vi "AI_snake.vi"() -> ()   [LabVIEW 2020]
uses:
  Typedef/Snake_states.ctl
panel:
  in  "speed":dbl=700.0 format="%#_13g"
  in  "level":dbl(slide) scale=1.0..5.0
  out "Stop Variable":bool
  out "Score":i32
  out "Snake Field":u32[][](array[colorbox])=[[0, 0, 0, 0, 0, 0, 0, 0, 0, 0, 0, 0, 0, 0, 0, 0, 0, 0, 0, 0, 0, 0, 0, 0, 0, 0, 0], [0, 0, 0, 0, 0, 0, 0, 0, 0, 0, 0, 0, 0, 0, 0, 0, 0, 0, 0, 0, 0, 0, 0, 0, 0, 0, 0], [0, 0, 0, 3622, 0, 0, 0, 0, 0, 0, 0, 0, 0, 0, 0, 0, 0, 0, 0, 0, 0, 0, 0, 0, 0, 0, 0], [0, 0, 0, 0, 0, 0, 0, 0, 0, 0, 0, 0, 0, 0, 0, 0, 0, 0, 0, 0, 0, 0, 0, 0, 0, 0, 0], [0, 0, 0, 0, 0, 0, 0, 0, 0, 0, 0, 0, 0, 0, 0, 0, 0, 0, 0, 0, 0, 0, 0, 0, 0, 0, 0], [0, 0, 0, 0, 0, 0, 0, 0, 0, 0, 0, 0, 0, 0, 0, 0, 0, 0, 0, 0, 0, 0, 0, 0, 0, 0, 0], [0, 0, 0, 0, 0, 0, 0, 0, 0, 0, 0, 0, 0, 0, 0, 0, 0, 0, 0, 0, 0, 0, 0, 0, 0, 0, 0], [0, 0, 0, 0, 0, 0, 0, 0, 0, 0, 0, 0, 0, 0, 0, 0, 0, 0, 0, 0, 0, 0, 0, 0, 0, 0, 0], [0, 0, 0, 0, 0, 0, 0, 0, 0, 0, 0, 0, 0, 0, 0, 0, 0, 0, 0, 0, 0, 0, 0, 0, 0, 0, 0], [0, 0, 0, 0, 0, 0, 0, 0, 0, 0, 0, 0, 0, 0, 0, 0, 0, 0, 0, 0, 0, 0, 0, 0, 0, 0, 0], [0, 0, 0, 0, 0, 0, 0, 0, 0, 0, 0, 0, 0, 0, 0, 0, 0, 0, 0, 0, 0, 0, 0, 0, 0, 0, 0], [0, 0, 0, 0, 0, 0, 0, 0, 0, 0, 0, 0, 0, 0, 0, 0, 0, 0, 0, 0, 0, 0, 0, 0, 0, 0, 0], [0, 0, 0, 0, 0, 0, 0, 0, 0, 0, 0, 0, 0, 0, 0, 0, 0, 0, 0, 0, 0, 0, 0, 0, 0, 0, 0], [0, 0, 0, 0, 0, 0, 0, 0, 0, 0, 0, 0, 0, 0, 0, 0, 0, 0, 0, 0, 0, 0, 0, 0, 0, 0, 0], [0, 0, 0, 0, 0, 0, 0, 0, 0, 0, 0, 0, 0, 0, 0, 0, 0, 0, 0, 0, 0, 0, 0, 0, 0, 0, 0], [0, 0, 0, 0, 0, 0, 0, 0, 0, 0, 0, 0, 0, 0, 0, 0, 0, 0, 0, 0, 0, 0, 0, 0, 0, 0, 0], [0, 0, 0, 0, 0, 0, 0, 0, 0, 0, 0, 0, 0, 0, 0, 0, 0, 0, 0, 0, 0, 0, 0, 0, 0, 0, 0], [0, 0, 0, 0, 0, 0, 0, 0, 0, 0, 0, 0, 0, 0, 0, 0, 0, 0, 0, 0, 0, 0, 0, 0, 0, 0, 0], [0, 0, 0, 0, 0, 0, 0, 0, 0, 0, 0, 0, 0, 0, 0, 0, 0, 0, 0, 0, 0, 0, 0, 0, 0, 0, 0], [0, 0, 0, 0, 0, 0, 0, 0, 0, 0, 0, 0, 0, 0, 0, 0, 0, 0, 0, 0, 0, 0, 0, 0, 0, 0, 0]]
  out "Y Direction":i32
  out "X Direction":i32
  in  "Stop":bool
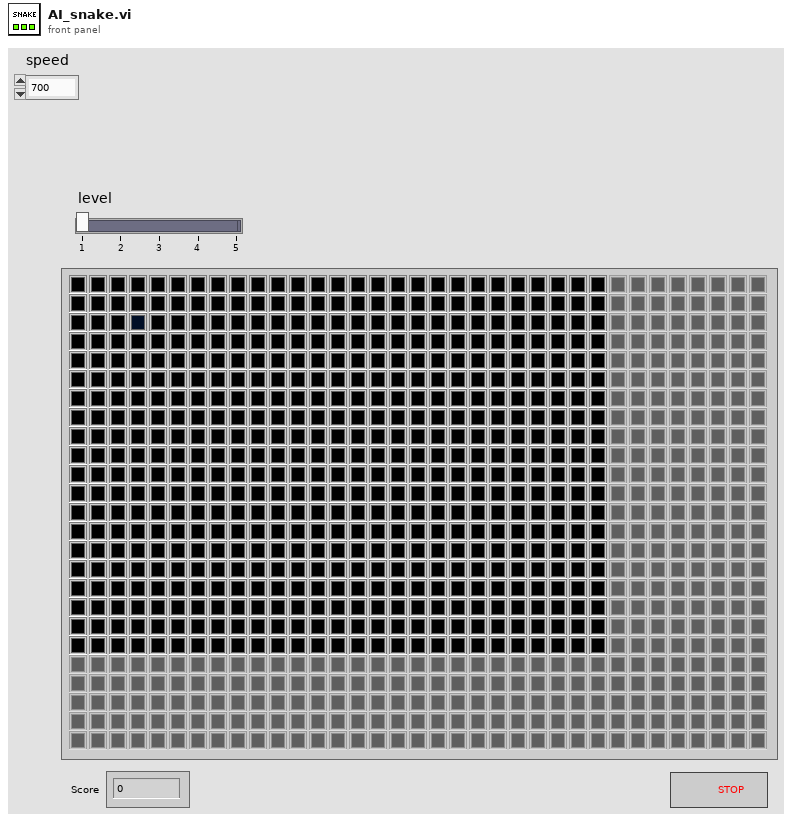
[diagram p1: front panel]
types:
  T1 = typedef "Snake_states.ctl" = enum16{"Initialize", "Start game", "Wait for user to press button", "Stop"}
  T2 = typedef "eventvkey.ctl" = enum16{"ASCII", "Enter", "Return", "Shift", "Ctrl", "Alt", "Cmd", "Opt", "Caps", "NumLock", "Clear", "Break", "Up", "Down", "Left", "Right", "Insert", "Delete", "Home", "End", "PageUp", "PageDown", "Escape", "Help", "Pause", "ScrollLock", "F1", "F2", "F3", "F4", "F5", "F6", "F7", "F8", "F9", "F10", "F11", "F12", "F13", "F14", "F15", "F16", "F17", "F18", "F19", "F20", "F21", "F22", "F23", "F24", "Play", "VolumeUp", "VolumeDown", "Mute", "Two Byte Char"}
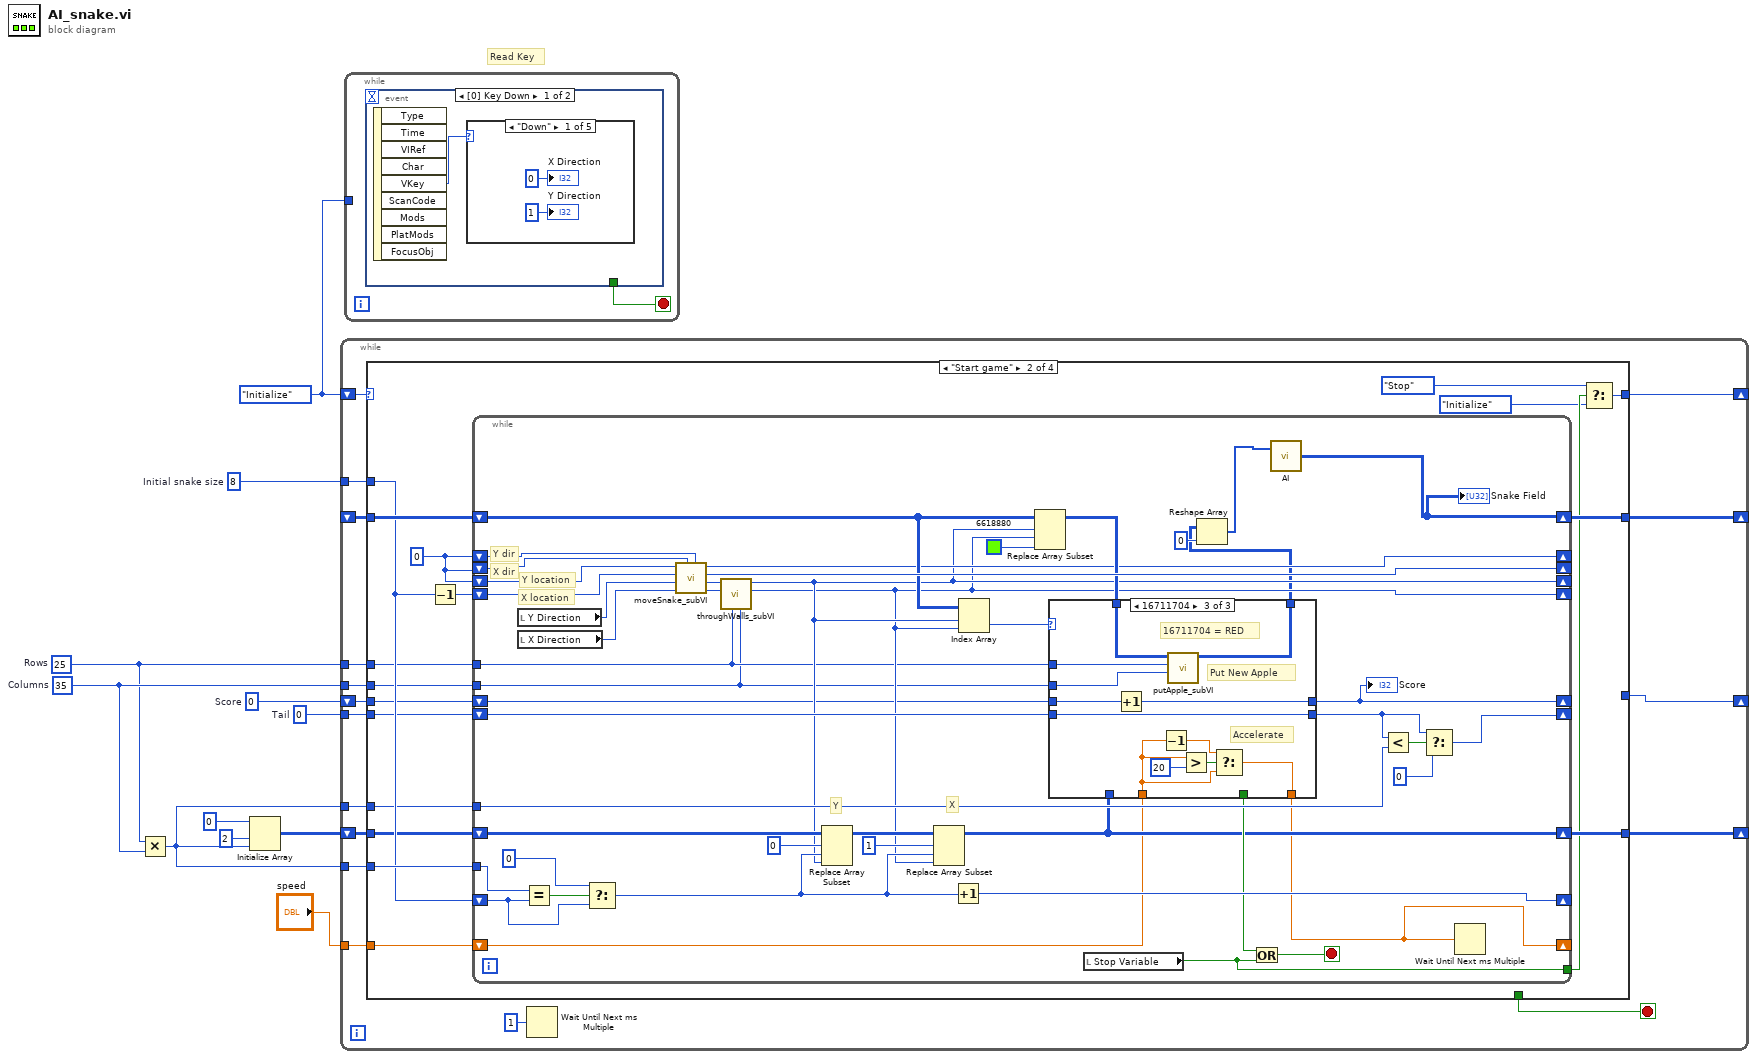
[diagram p0: block diagram]
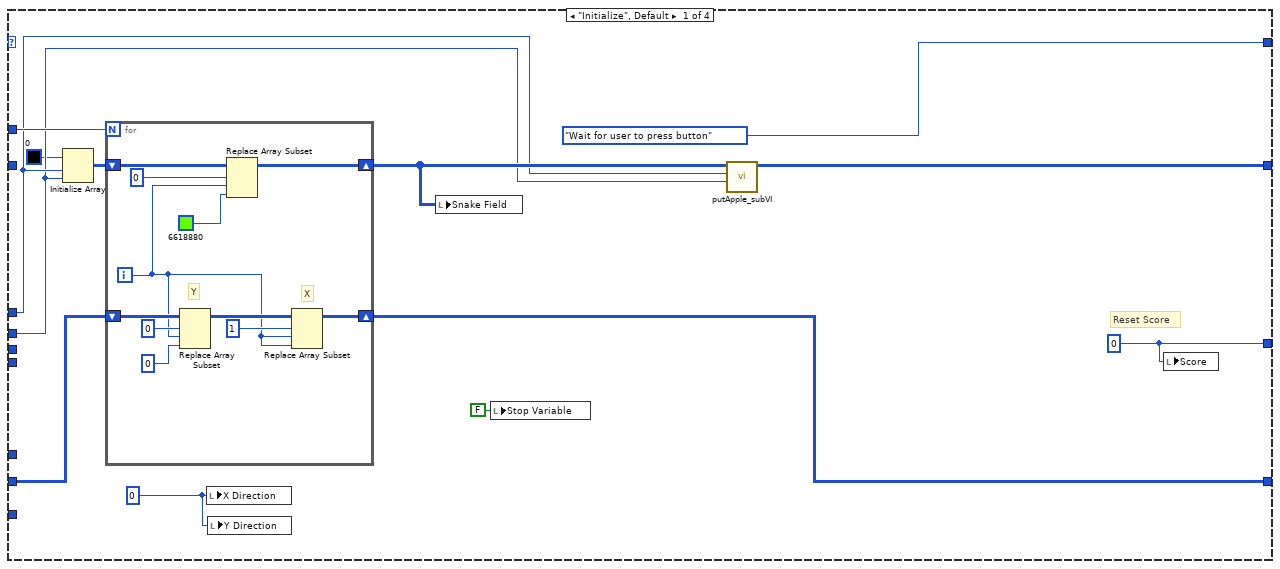
[diagram p2: hidden frame]
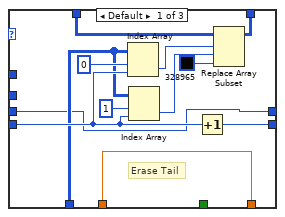
[diagram p3: hidden frame]
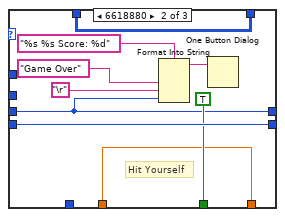
[diagram p4: hidden frame]
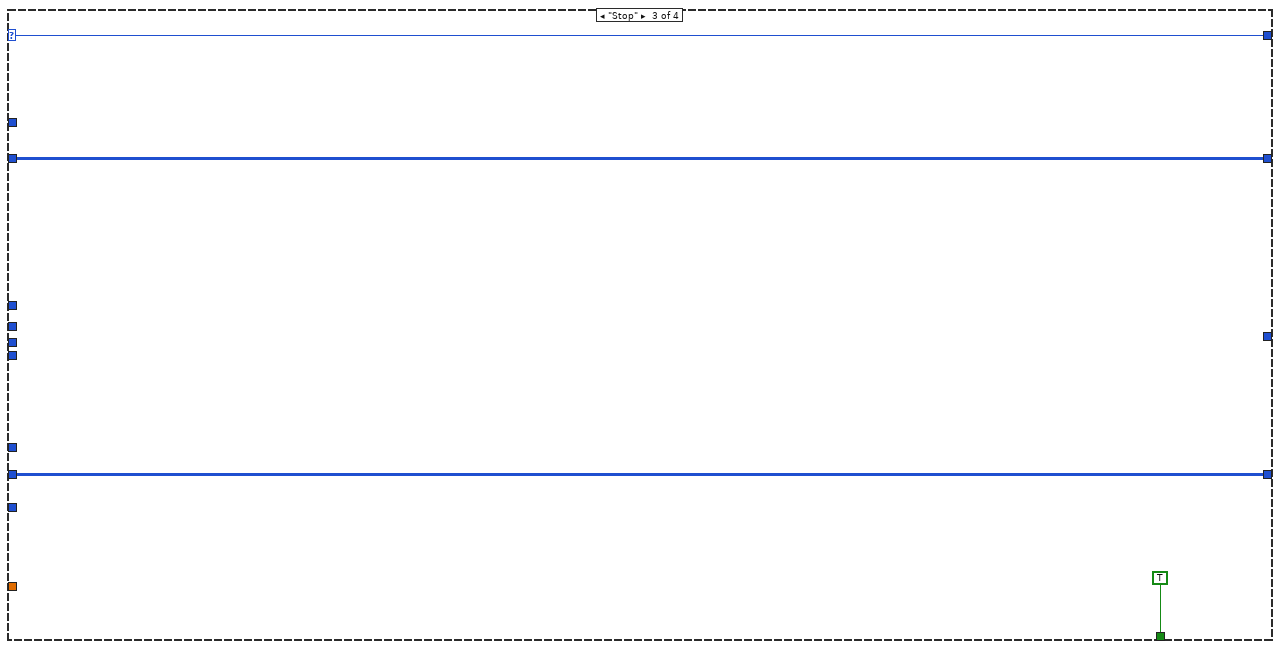
[diagram p5: hidden frame]
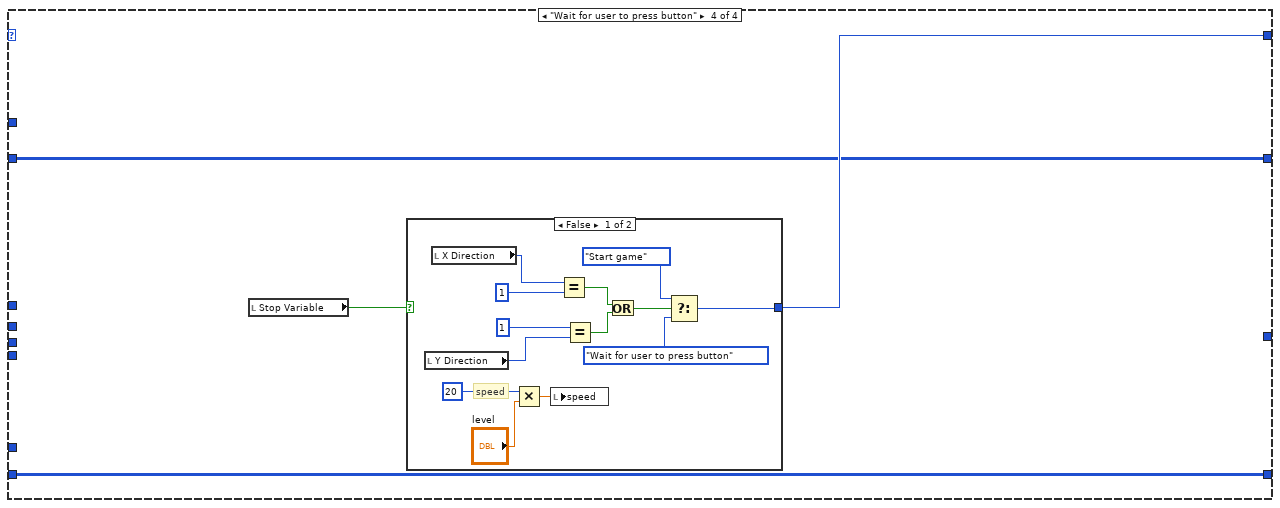
[diagram p6: hidden frame]
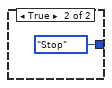
[diagram p7: hidden frame]
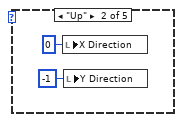
[diagram p8: hidden frame]
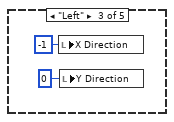
[diagram p9: hidden frame]
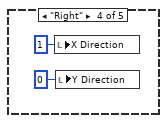
[diagram p10: hidden frame]
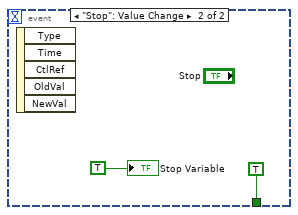
[diagram p12: hidden frame]
diagram:
  w2 = 0  # Score
  w6 = 0  # Tail
  w10 = 8  # Initial snake size
  w5 = 35  # Columns
  w4 = 25  # Rows
  w11 = Snake_states."Initialize"
  # "Read Key"
  n1 = Multiply(x=w4, y=w5) -> (x*y=w3:i32)
  n2 = Initialize Array(0 ("element"), 2 ("dimension size"), w3) -> (w7:i32[][])
  n3 = while {
    shift-right: [w27] -> _
    shift-left: w11 -> [w28]
    tunnel: w3 -> [w25]
    tunnel: w10 -> [w24]
    shift-right: [w23] -> _
    shift-left: _ -> [w26]
    shift-right: [w21] -> _
    shift-left: w7 -> [w22]
    tunnel: w6 -> [w20]
    tunnel: w5 -> [w19]
    tunnel: w4 -> [w18]
    tunnel: w3 -> [w17]
    shift-right: [w14] -> _
    shift-left: w2 -> [w15]
    tunnel: "speed" -> [w13]
    stop <- w16 stop-if-true
    n4 = case shown="\"Start game\"" w28 {
      selector: w28 -> [_ _ w153 _]
      tunnel: [Snake_states."Wait for user to press button" w59 w153 w157] -> w27
      tunnel: w26 -> [_ w70 w152 w156]
      tunnel: w25 -> [_ w69 _ _]
      tunnel: w24 -> [w39 w66 _ _]
      tunnel: [w35 w68 w152 w156] -> w23
      tunnel: w22 -> [w38 w65 w151 w155]
      tunnel: [w37 w64 w151 w155] -> w21
      tunnel: w18 -> [w34 w63 _ _]
      tunnel: w19 -> [w33 w62 _ _]
      tunnel: w20 -> [_ w61 _ _]
      tunnel: w17 -> [_ w60 _ _]
      tunnel: [_ _ TRUE _] -> w16
      tunnel: w15 -> [_ w54 _ _]
      tunnel: [w30 _ _ _] -> w14
      tunnel: w13 -> [_ w53 _ _]
      frame "Initialize", Default {
        w30 = 0 ("index (row)")
        w40 = 0 ("X Direction")
        # "Reset Score"
        n5 = Initialize Array(u32 0 ("Color Box"), w34, w33) -> (w31:u32[][])
        n6 = for {
          N: w39 -> [_]
          shift-right: [w49] -> w36
          shift-left: w31 -> [w51]
          shift-right: [w42] -> w37
          shift-left: w38 -> [w47]
          i -> [w43]
          # "X"
          # "Y"
          n7 = Replace Array Subset(array=w47, new element=0 ("new element/subarray"), index (row)=0, index (col)=w43) -> (w46:i32[][])
          n8 = Replace Array Subset(array=w51, new element=u32 6618880 ("Color Box"), index (row)=0, index (col)=w43) -> (w49:u32[][])
          n9 = Replace Array Subset(array=w46, new element=w43, index (row)=1, index (col)=w43) -> (w42:i32[][])
        }
        n10 = local write "X Direction"(w40) -> ()
        n11 = local write "Y Direction"(w40) -> ()
        n12 = local write "Snake Field"(w36) -> ()
        n13 = local write "Stop Variable"(FALSE ("Stop Variable")) -> ()
        n14 = call "putApple_subVI.vi"("Field Width"=w33, "Field Height"=w34, "Snake Field in"=w36) -> ("Snake Field out"=w35:u32[][])  [unwired: 8 in]
        n15 = local write "Score"(w30) -> ()
      }
      frame "Start game" {
        w55 = 0 ("Current Direction Y")
        n16 = Decrement(x=w66) -> (x-1=w67:i32)
        n17 = while {
          shift-right: [w84] -> _
          shift-left: w55 -> [w116]
          shift-right: [w83] -> _
          shift-left: w67 -> [w115]
          shift-right: [w71] -> w68
          shift-left: w70 -> [w97]
          tunnel: w69 -> [w110]
          shift-right: [w111] -> _
          shift-left: w66 -> [w107]
          shift-right: [w80] -> w64
          shift-left: w65 -> [w106]
          tunnel: w63 -> [w82]
          tunnel: w62 -> [w81]
          shift-right: [w87] -> _
          shift-left: w55 -> [w100]
          shift-right: [w101] -> _
          shift-left: w55 -> [w99]
          shift-right: [w91] -> _
          shift-left: w61 -> [w96]
          tunnel: w60 -> [w95]
          tunnel: [w75] -> w58
          shift-right: [w78] -> _
          shift-left: w54 -> [w79]
          shift-right: [w76] -> _
          shift-left: w53 -> [w77]
          stop <- w89 stop-if-true
          # "X location"
          # "Y location"
          # "X dir"
          # "Y dir"
          # "X"
          # "Y"
          n18 = local read "Y Direction"() -> (w114:i32)
          n19 = local read "X Direction"() -> (w113:i32)
          n20 = Equal?(x=w110, y=w107) -> (x = y?=w109:bool)
          n21 = Select(t=0, s=w109, f=w107) -> (s? t:f=w102:i32)
          n22 = call "moveSnake_subVI.vi"("Old Direction Y"=w100, "Old Direction X"=w99, "New Direction X"=w113, "New Direction Y"=w114, "Snake Head X"=w115, "Snake Head Y"=w116) -> ("New Snake Head X"=w85:i32, "New Snake Head Y"=w86:i32, "Current Direction X"=w101:i32, "Current Direction Y"=w87:i32)  [unwired: 2 in]
          n23 = call "throughWalls_subVI.vi"("Columns"=w81, "Rows"=w82, "Next X"=w85, "Next Y"=w86) -> ("Next X"=w83:i32, "Next Y"=w84:i32)  [unwired: 6 in]
          n24 = Replace Array Subset(array=w106, new element=w84, index (row)=0, index (col)=w102) -> (w105:i32[][])
          n25 = Replace Array Subset(array=w105, new element=w83, index (row)=1, index (col)=w102) -> (w80:i32[][])
          n26 = Increment(x=w102) -> (x+1=w111:i32)
          n27 = Index Array(array=w97, index (row)=w84, index (col)=w83) -> (element=w90:u32)
          n28 = Replace Array Subset(array=w97, new element=u32 6618880 ("Color Box"), index (row)=w84, index (col)=w83) -> (w98:u32[][])
          n29 = case shown="16711704" w90 {
            tunnel: w82 -> [_ _ w148]
            tunnel: w81 -> [_ _ w147]
            tunnel: w98 -> [w128 w137 w149]
            tunnel: [w127 w137 w146] -> w72
            tunnel: w96 -> [w121 w136 w145]
            tunnel: [w120 w136 w145] -> w93
            tunnel: [_ TRUE _] -> w88
            tunnel: w80 -> [w119 _ _]
            tunnel: w79 -> [w118 w131 w144]
            tunnel: [w118 w131 w143] -> w78
            tunnel: w77 -> [w117 w129 w138]
            tunnel: [w117 w129 w139] -> w76
            frame Default {
              # "Erase Tail"
              n30 = Index Array(array=w119, index (row)=0 ("disabled index (row)"), index (col)=w121) -> (element=w122:i32)
              n31 = Index Array(array=w119, index (row)=1, index (col)=w121) -> (element=w125:i32)
              n32 = Increment(x=w121) -> (x+1=w120:i32)
              n33 = Replace Array Subset(array=w128, new element=u32 328965 ("Color Box"), index (row)=w122, index (col)=w125) -> (w127:u32[][])
            }
            frame 6618880 {
              # "Hit Yourself"
              n34 = Format Into String(format string="%s %s Score: %d", "Game Over", "\r", w131) -> (resulting string=w132:string)  [unwired: 2 in, 1 out]
              n35 = One Button Dialog(message=w132) -> ()  [unwired: 1 in, 1 out]
            }
            frame 16711704 {
              # "Accelerate"
              # "16711704 = RED"
              # "Put New Apple"
              n36 = Increment(x=w144) -> (x+1=w143:i32)
              n37 = Decrement(x=w138) -> (x-1=w140:dbl)
              n38 = call "putApple_subVI.vi"("Field Width"=w147, "Field Height"=w148, "Snake Field in"=w149) -> ("Snake Field out"=w146:u32[][])  [unwired: 8 in]
              n39 = Greater?(x=w138, y=u32 20) -> (0:w141:bool)
              n40 = Select(t=w140, s=w141, f=w138) -> (s? t:f=w139:dbl)
            }
          }
          "Score" <- w78
          n41 = local read "Stop Variable"() -> (w75:bool)
          n42 = Reshape Array(w72, 0 ("dimension size")) -> (w73:u32[])
          n43 = Or(x=w88, y=w75) -> (x .or. y?=w89:bool)
          n44 = call "AI.vi"("input array"=w73) -> ("output array"=w71:u32[][])  [unwired: 1 in]
          "Snake Field" <- w71
          n45 = Less?(x=w93, y=w95) -> (x < y?=w94:bool)
          n46 = Select(t=w93, s=w94, f=0) -> (s? t:f=w91:i32)
          n47 = Wait Until Next ms Multiple(millisecond multiple=w76) -> ()  [unwired: 1 out]
        }
        n48 = Select(t=Snake_states."Stop", s=w58, f=Snake_states."Initialize") -> (s? t:f=w59:T1)
      }
      frame "Stop" {
      }
      frame "Wait for user to press button" {
        n49 = local read "Stop Variable"() -> (w154:bool)
        n50 = case shown="False" w154 {
          tunnel: [w161 Snake_states."Stop"] -> w157
          frame False {
            # "speed"
            n51 = local read "Y Direction"() -> (w170:i32)
            n52 = local read "X Direction"() -> (w168:i32)
            n53 = Multiply(x=u32 20 ("Speed"), y="level") -> (x*y=w160:dbl)
            n54 = local write "speed"(w160) -> ()
            n55 = Equal?(x=w168, y=1) -> (x = y?=w165:bool)
            n56 = Equal?(x=1, y=w170) -> (x = y?=w166:bool)
            n57 = Or(x=w165, y=w166) -> (x .or. y?=w164:bool)
            n58 = Select(t=Snake_states."Start game", s=w164, f=Snake_states."Wait for user to press button") -> (s? t:f=w161:T1)
          }
          frame True {
          }
        }
      }
    }
    n59 = Wait Until Next ms Multiple(millisecond multiple=u32 1) -> ()  [unwired: 1 out]
  }
  n60 = while {
    tunnel: w11 -> [_]
    stop <- w172 stop-if-true
    n61 = event shown="[0] Key Down" {
      selector: _ -> [_ _]
      dyn-events: _ -> [_ _]
      timeout: _ -> [_ _]
      tunnel: [_ TRUE] -> w172
      event Key Down {
        n62 = event-data() -> ("VKey"=w173:T2)  [unwired: 1 in, 8 out]
        n63 = case shown="\"Down\"" w173 {
          frame "Down" {
            "X Direction" <- 0 ("X Direction")
            "Y Direction" <- 1 ("Y Direction")
          }
          frame "Up" {
            n64 = local write "X Direction"(0 ("X Direction")) -> ()
            n65 = local write "Y Direction"(-1 ("Y Direction")) -> ()
          }
          frame "Left" {
            n66 = local write "X Direction"(-1 ("X Direction")) -> ()
            n67 = local write "Y Direction"(0 ("Y Direction")) -> ()
          }
          frame "Right" {
            n68 = local write "X Direction"(1 ("X Direction")) -> ()
            n69 = local write "Y Direction"(0 ("Y Direction")) -> ()
          }
          frame "End", Default {
          }
        }
      }
      event "Stop": Value Change {
        n70 = event-data() -> ()  [unwired: 1 in, 5 out]
        "Stop Variable" <- TRUE
      }
    }
  }
